vi "fgv_erp42_opval.vi"(7 "cmd":enum16{"read", "write", "ini"}(ring), 11 "data_in":T1={"Drive_value"={"F/B"=enum."Go", "Speed"=0, "Steer"=0, "A/M"=enum."Auto", "Brake"=0}} {"Drive_value"."Brake" scale=0.0..200.0; "Drive_value"."Steer" scale=-2000.0..2000.0; "Drive_value"."Speed" scale=0.0..100.0}) -> (3 "data_out":T1={"Drive_value"={"F/B"=enum."Go", "Speed"=0, "Steer"=0, "A/M"=enum."Auto", "Brake"=0}} {"Drive_value"."Brake" scale=0.0..200.0; "Drive_value"."Steer" scale=-2000.0..2000.0; "Drive_value"."Speed" scale=0.0..100.0})   [LabVIEW 2019]
uses:
  Ctrl/data.ctl
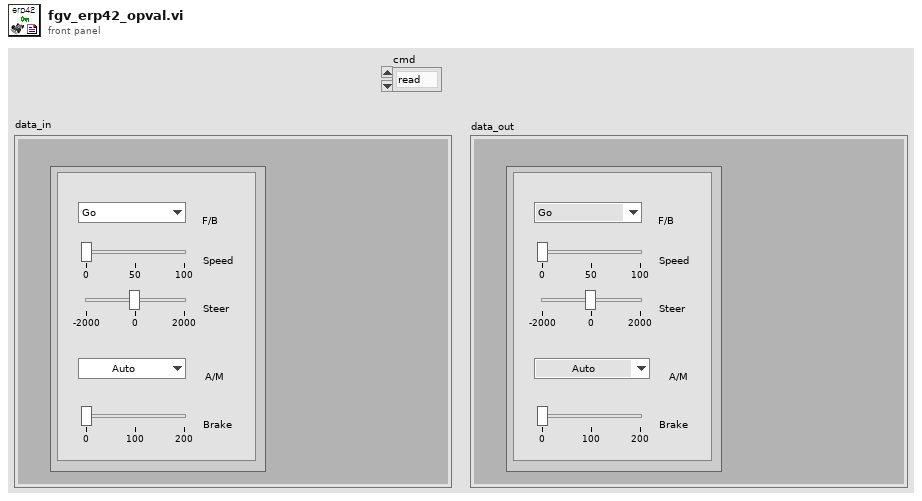
[diagram p1: front panel]
types:
  T1 = typedef "data.ctl" = cluster{"Drive_value":cluster{"F/B":enum16{"Go", "N", "Back"}, "Speed":u16, "Steer":i16, "A/M":enum16{"Brake", "Auto", "Manual"}, "Brake":u8}}
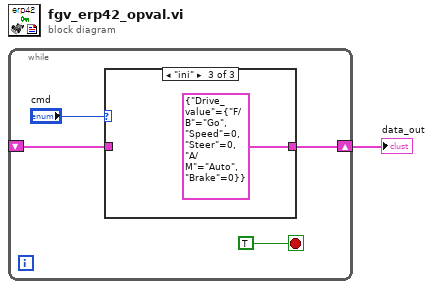
[diagram p0: block diagram]
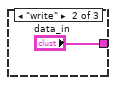
[diagram p3: hidden frame]
diagram:
  n1 = while {
    shift-right: [w3] -> w1
    shift-left: _ -> [w2]
    stop <- TRUE stop-if-true
    n2 = case shown="\"ini\"" "cmd" {
      tunnel: [w6 "data_in" T1 {"Drive_value"={"F/B"=enum."Go", "Speed"=0, "Steer"=0, "A/M"=enum."Auto", "Brake"=0}} ("Data")] -> w3
      tunnel: w2 -> [w6 _ _]
      frame "read", Default {
      }
      frame "write" {
      }
      frame "ini" {
      }
    }
  }
  "data_out" <- w1
